vi "Email_With_Log.vi"(0 "recipients":string[](array[string]), 1 "subject ([No Subject])":string="[No Subject]", 2 "message":string, 3 "attachments":path[](array[path])) -> (5 "invalid recipients":string[](array[string]), 6 "error out":errorcluster)   [LabVIEW 2022 SP3]
uses:
  272fa2c8-f8d7-1949-8157-cfb0dd8301bf.vi
  Globals/Preference_global.vi
  Globals/Constants_global.vi
panel:
  out "Number of valid email requests":i32
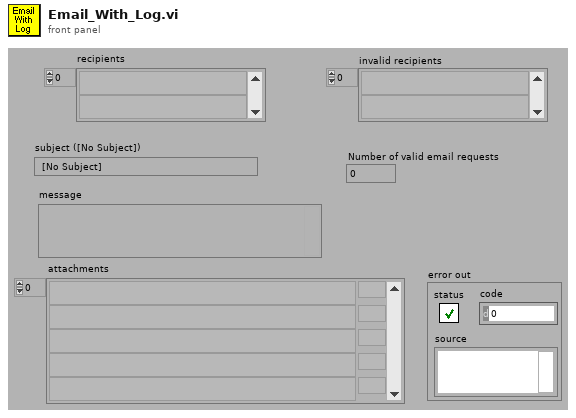
[diagram p1: front panel]
types:
  T1 = typedef "SMTPCredentials.ctl" = cluster{"User Name":string, "Password":string, "Reply to Address":string, "From Domain":string}
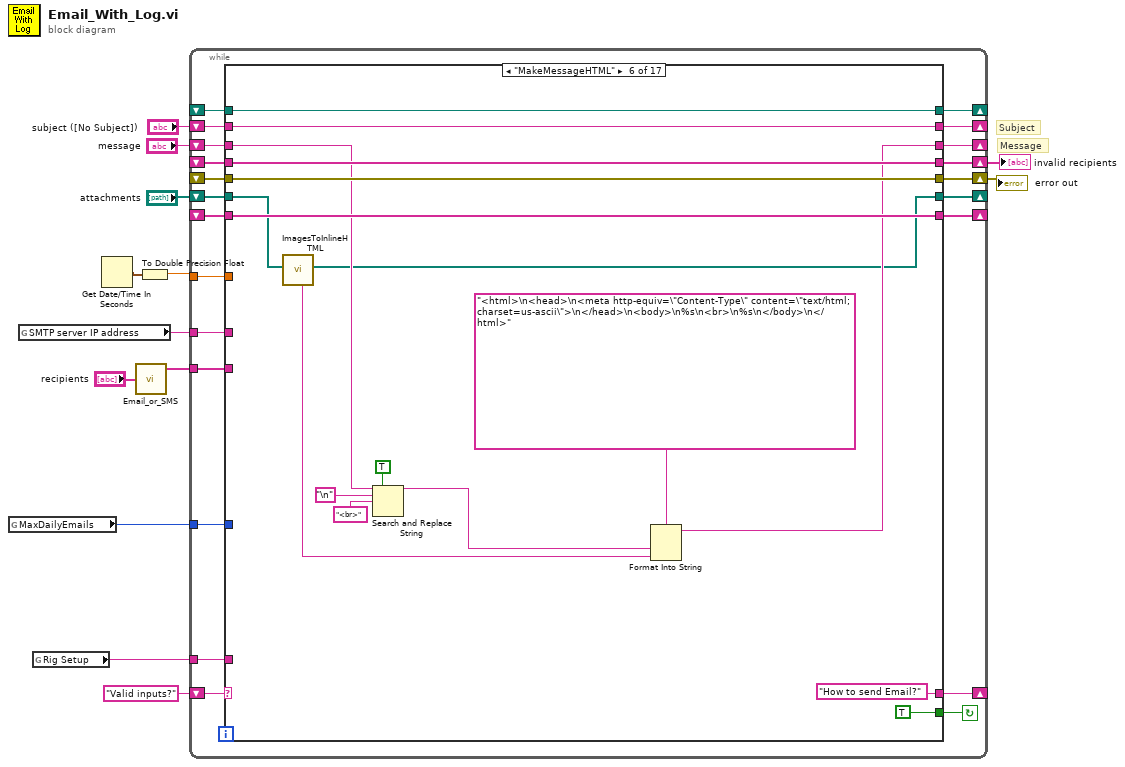
[diagram p0: block diagram]
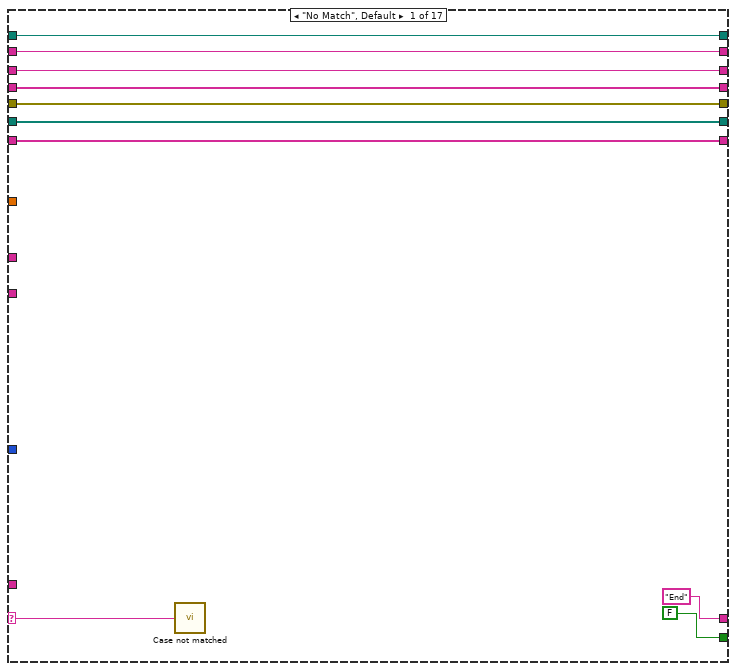
[diagram p2: hidden frame]
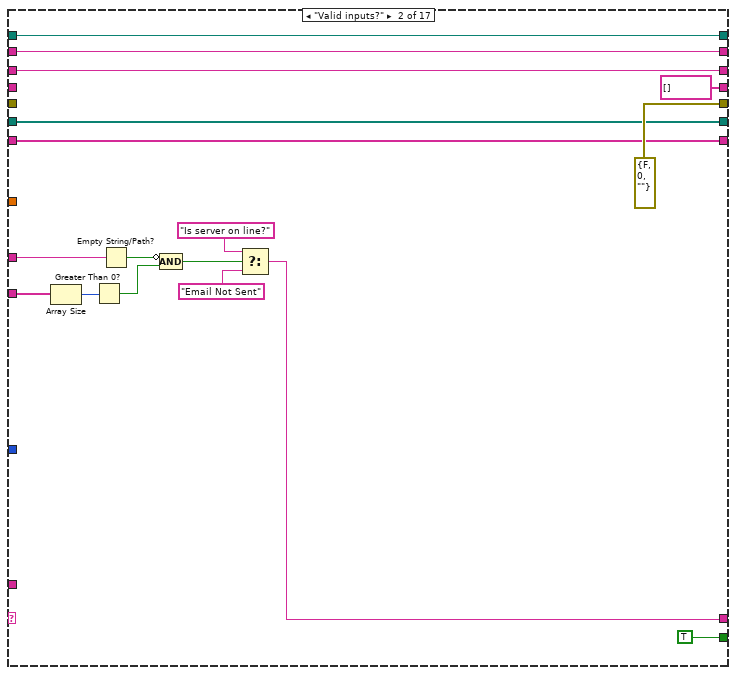
[diagram p3: hidden frame]
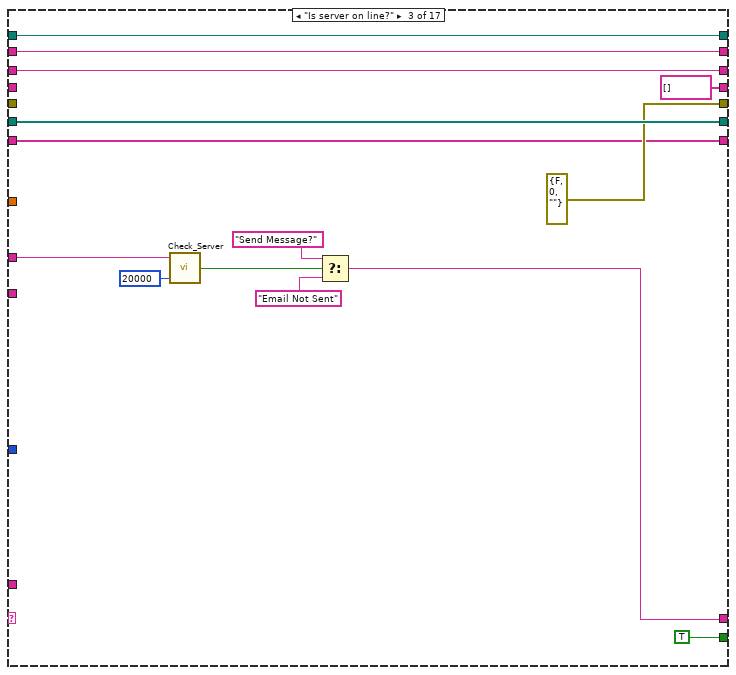
[diagram p4: hidden frame]
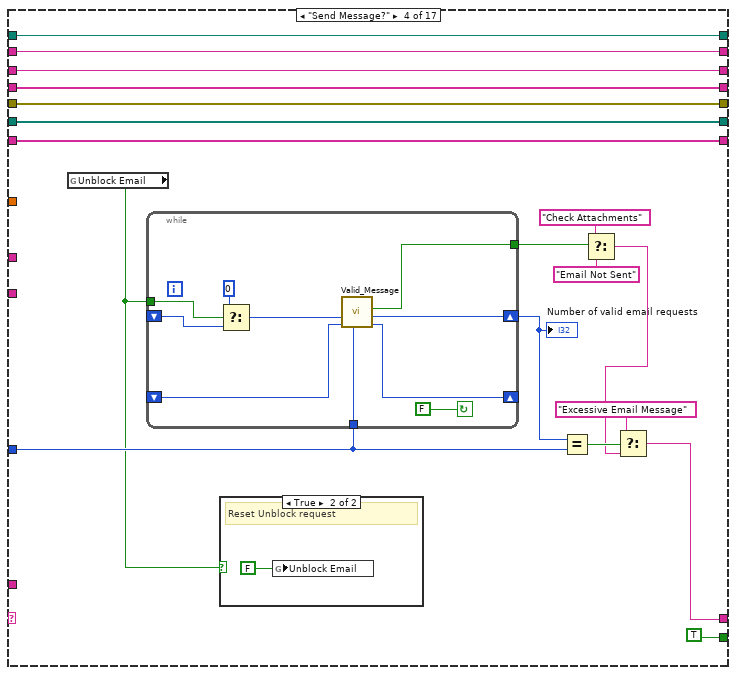
[diagram p5: hidden frame]
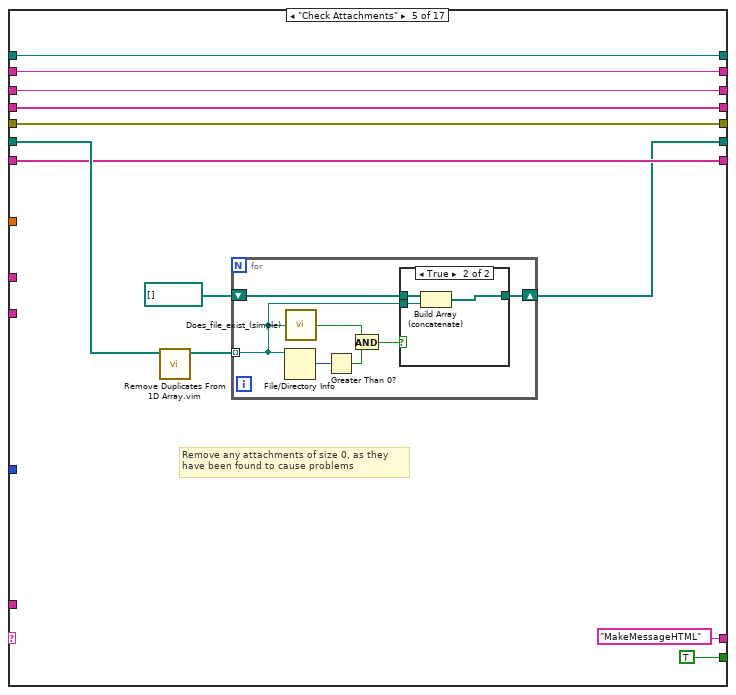
[diagram p7: hidden frame]
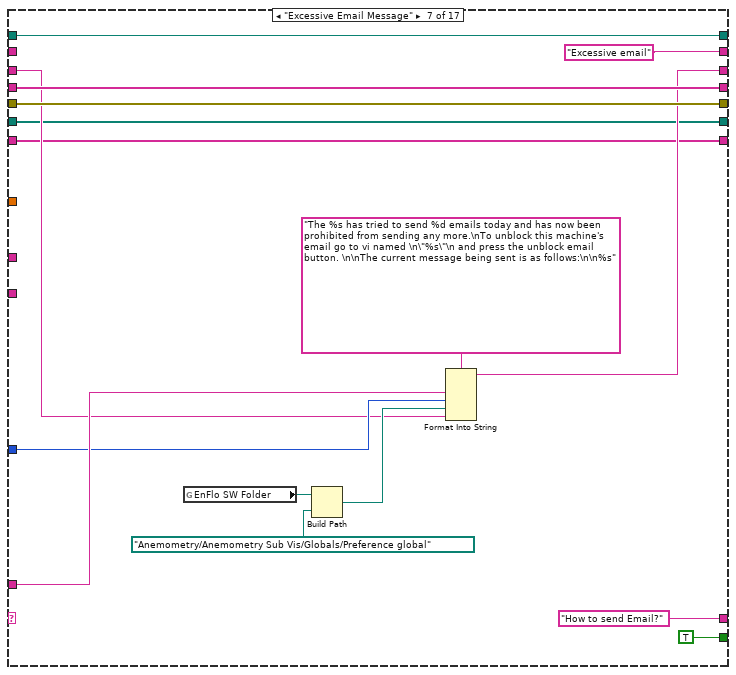
[diagram p9: hidden frame]
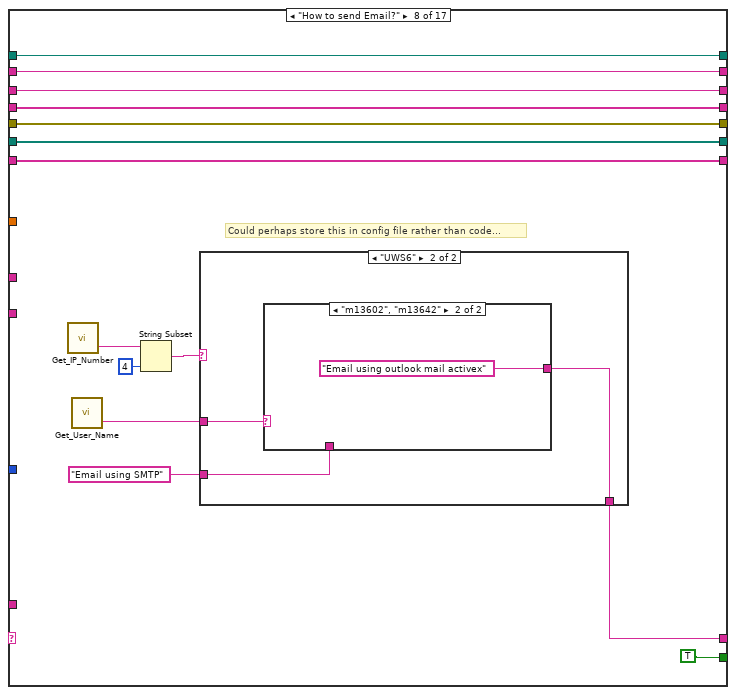
[diagram p10: hidden frame]
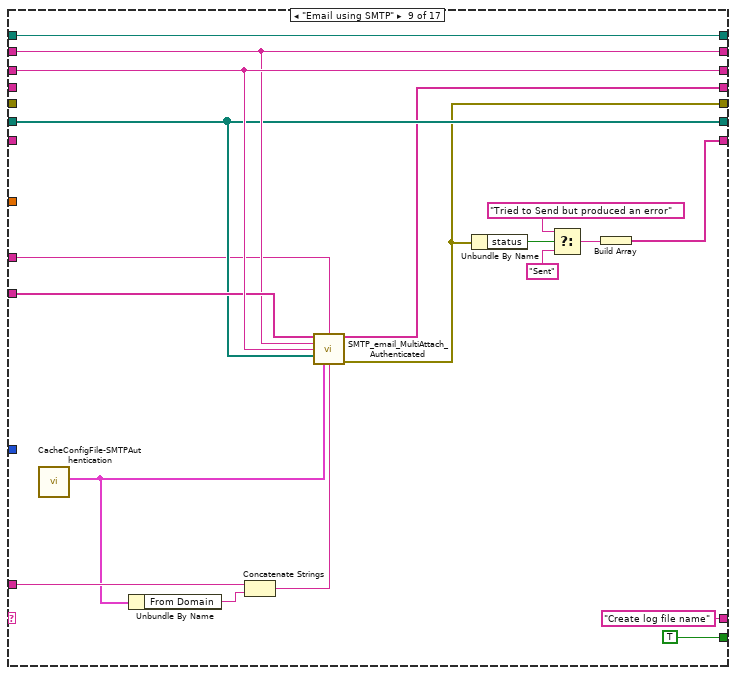
[diagram p13: hidden frame]
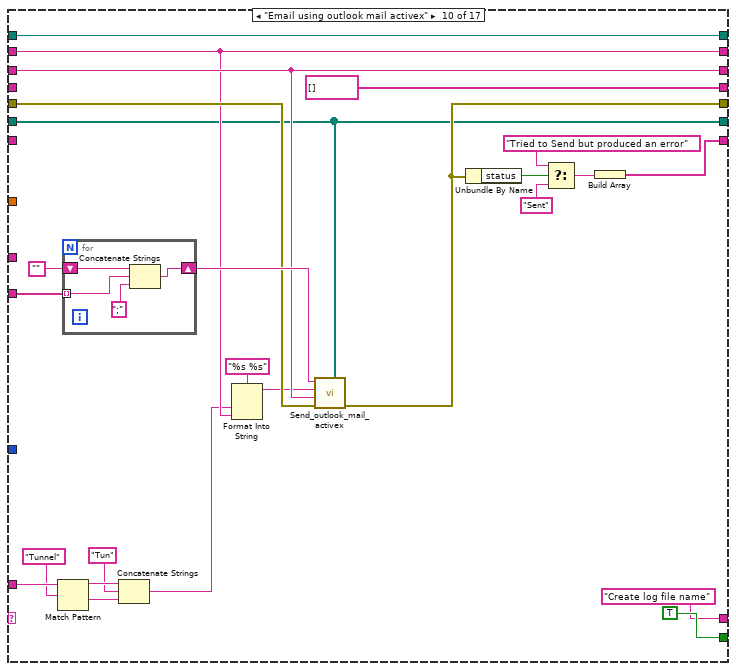
[diagram p14: hidden frame]
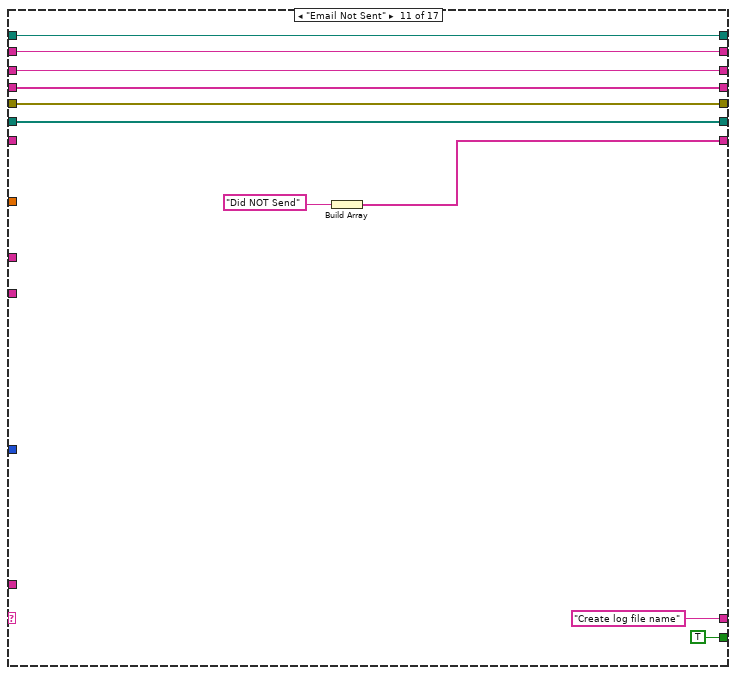
[diagram p15: hidden frame]
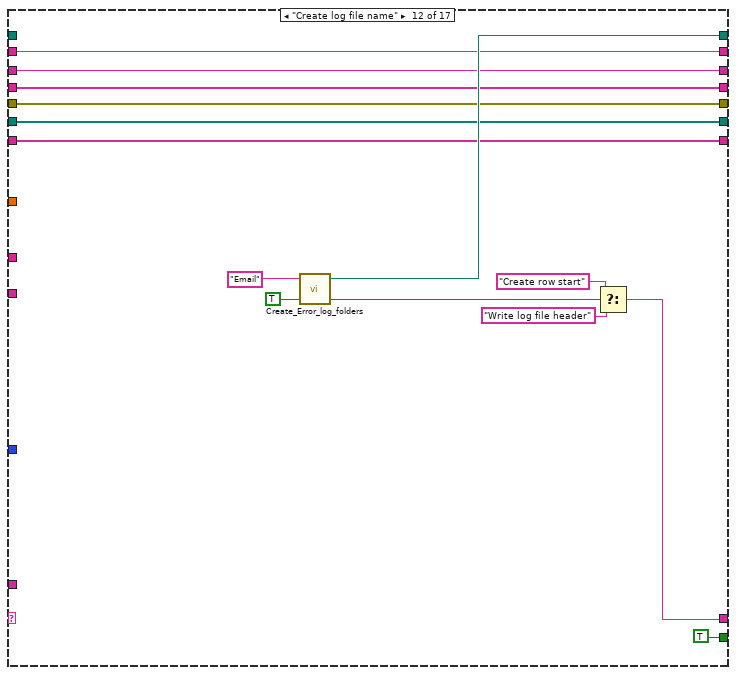
[diagram p16: hidden frame]
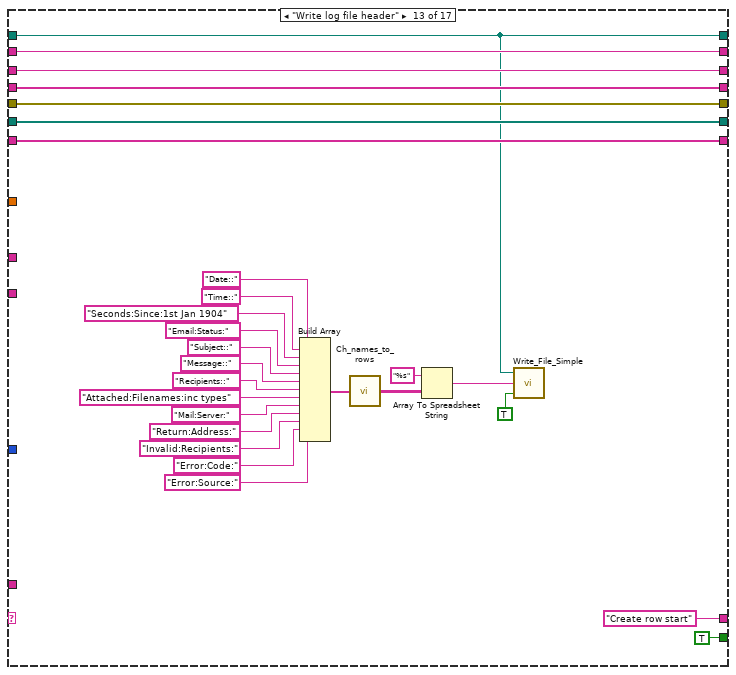
[diagram p17: hidden frame]
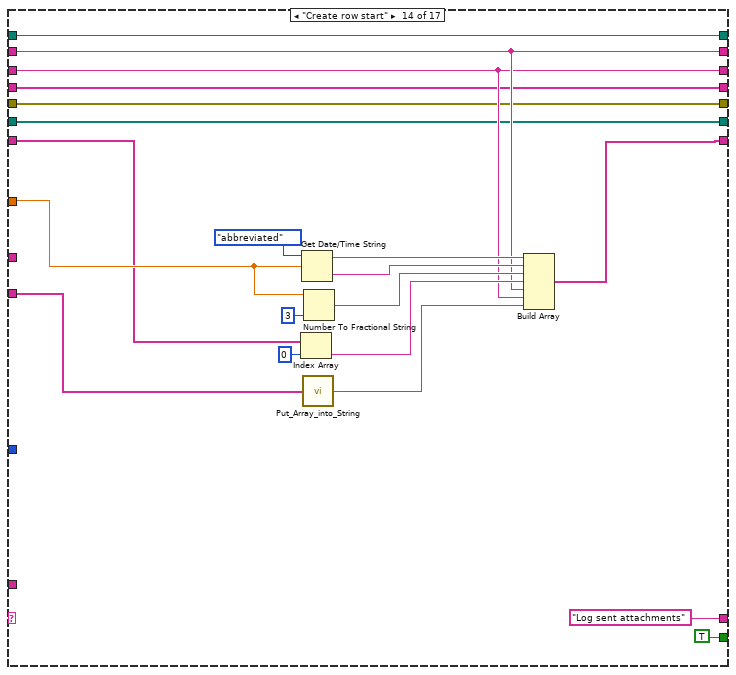
[diagram p18: hidden frame]
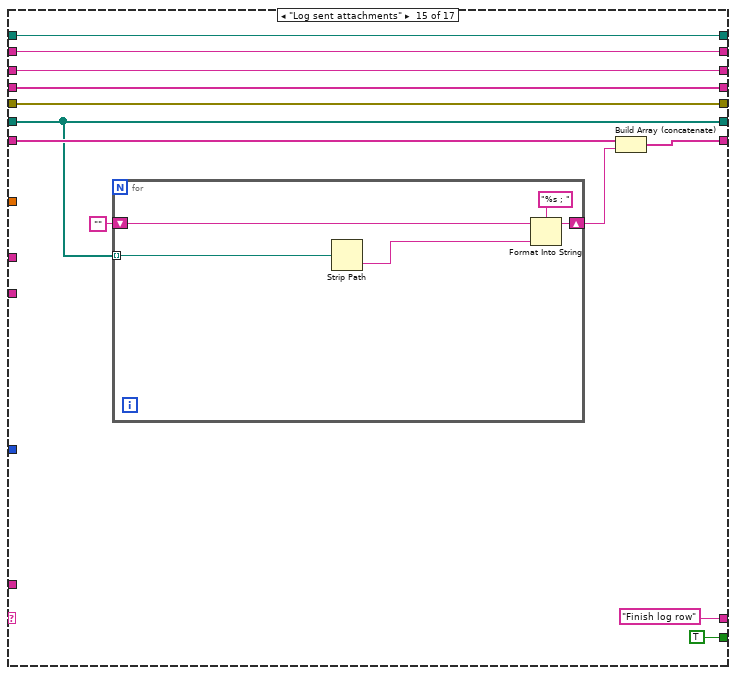
[diagram p19: hidden frame]
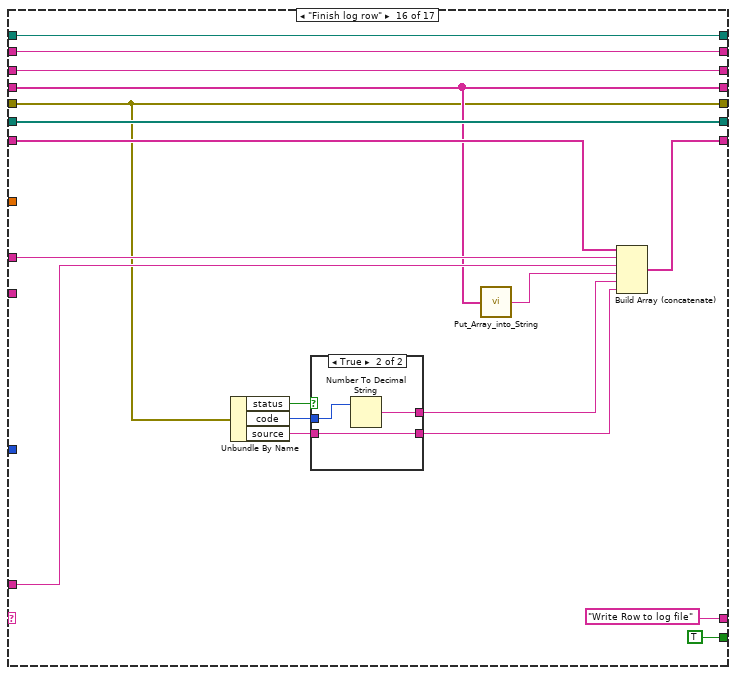
[diagram p20: hidden frame]
diagram:
  # "Message"
  # "Subject"
  n1 = global read "Preference_global.vi" "MaxDailyEmails"() -> (w1:u32)
  n2 = global read "Preference_global.vi" "SMTP server IP address"() -> (w4:string)
  n3 = global read "Preference_global.vi" "Rig Setup"() -> (w2:string)
  n4 = Get Date/Time In Seconds() -> (seconds since 1Jan1904=w12:timestamp)
  n5 = call "Email_or_SMS.vi"("Email address"="recipients") -> ("Email"=w5:string[])  [unwired: 3 out]
  n6 = To Double Precision Float(number=w12) -> (double precision float=w13:dbl)
  n7 = while {
    tunnel: w13 -> [w33]
    shift-left: "Valid inputs?" -> [w32]
    shift-right: [w34] -> _
    shift-right: [w30] -> _
    shift-left: _ -> [w31]
    tunnel: w1 -> [w29]
    shift-right: [w27] -> _
    shift-left: "subject ([No Subject])" -> [w28]
    shift-right: [w26] -> _
    shift-left: "message" -> [w25]
    shift-right: [w23] -> w9
    shift-left: _ -> [w24]
    shift-right: [w22] -> w3
    shift-left: _ -> [w21]
    tunnel: w2 -> [w20]
    shift-right: [w18] -> _
    shift-left: "attachments" -> [w19]
    tunnel: w5 -> [w17]
    tunnel: w4 -> [w16]
    shift-right: [w15] -> _
    shift-left: _ -> [w14]
    stop <- w35 continue-if-true
    n8 = case shown="\"MakeMessageHTML\"" w32 {
      selector: w32 -> [w36 _ _ _ _ _ _ _ _ _ _ _ _ _ _ _ _]
      tunnel: [FALSE ("Abort") TRUE ("Abort") TRUE ("Abort") TRUE ("Abort") TRUE ("Abort") TRUE ("Abort") TRUE ("Abort") TRUE ("Abort") TRUE ("Abort") TRUE ("Abort") TRUE ("Abort") TRUE ("status") TRUE TRUE TRUE TRUE FALSE] -> w35
      tunnel: ["End" ("f") w52 w70 w83 "MakeMessageHTML" ("f") "How to send Email?" ("f") "How to send Email?" ("f") w164 "Create log file name" ("f") "Create log file name" ("f") "Create log file name" ("f") w251 "Create row start" ("f") "Log sent attachments" ("f") "Finish log row" ("f") "Write Row to log file" ("f") "End" ("f")] -> w34
      tunnel: w33 -> [_ _ _ _ _ _ _ _ _ _ _ _ _ w295 _ _ _]
      tunnel: w31 -> [w43 w61 w75 w93 w116 w144 w160 w174 w199 w224 w238 _ w255 w292 w310 w333 w341]
      tunnel: [w43 w61 w75 w93 w116 w144 w160 w174 w199 w224 w238 w248 w255 w292 w310 w333 w341] -> w30
      tunnel: w29 -> [_ _ _ w91 _ _ w150 _ _ _ _ _ _ _ _ _ _]
      tunnel: w28 -> [w42 w48 w74 w90 w115 w143 _ w172 w195 w209 w237 w246 w268 w285 w308 w331 w348]
      tunnel: [w42 w48 w74 w90 w115 w143 "Excessive email" ("Email address") w172 w195 w209 w237 w246 w268 w285 w308 w331 w348] -> w27
      tunnel: [w41 w60 w73 w89 w114 w133 w154 w173 w198 w214 w236 w245 w267 w284 w307 w330 w347] -> w26
      tunnel: w25 -> [w41 w60 w73 w89 w114 w132 w149 w173 w198 w214 w236 w245 w267 w284 w307 w330 w347]
      tunnel: w24 -> [w40 _ _ w88 w113 w142 w159 w170 _ _ w235 w244 w266 w283 w306 w325 w346]
      tunnel: [w40 string[] [] ("invalid recipients") string[] [] ("invalid recipients") w88 w113 w142 w159 w170 w185 string[] [] ("invalid recipients") w235 w244 w266 w283 w306 w325 w346] -> w23
      tunnel: [w39 errorcluster {"status"=FALSE, "code"=0, "source"=""} ("error out") errorcluster {"status"=FALSE, "code"=0, "source"=""} ("error out") w87 w112 w141 w158 w169 w193 w212 w234 w243 w265 w282 w305 w323 w345] -> w22
      tunnel: w21 -> [w39 _ _ w87 w112 w141 w158 w169 _ w213 w234 w243 w265 w282 w305 w323 w345]
      tunnel: w20 -> [_ _ _ _ _ _ w153 _ w187 w207 _ _ _ _ _ w326 _]
      tunnel: w19 -> [w38 w46 w69 w79 w111 w131 w147 w171 w194 w201 w233 w242 w264 w281 w301 w329 w344]
      tunnel: [w38 w46 w69 w79 w106 w130 w147 w171 w194 w201 w233 w242 w264 w281 w301 w329 w344] -> w18
      tunnel: w17 -> [_ w59 _ _ _ _ _ _ w197 w216 _ _ _ w287 _ _ _]
      tunnel: w16 -> [_ w57 w65 _ _ _ _ _ w184 _ _ _ _ _ _ w327 _]
      tunnel: w14 -> [w37 w50 w67 w78 w109 w139 w146 w168 _ _ _ w241 w257 w291 w302 w328 w343]
      tunnel: [w37 w50 w67 w78 w109 w139 w146 w168 w188 w218 w230 w241 w257 w288 w309 w332 w343] -> w15
      frame "No Match", Default {
        n9 = call "Case not matched.vi"("Case Name not Matched"=w36) -> ()
      }
      frame "Valid inputs?" {
        n10 = Array Size(array=w59) -> (size(s)=w58:i32)
        n11 = Greater Than 0?(x=w58) -> (x > 0?=w56:bool)
        n12 = Empty String/Path?(string/path=w57) -> (empty?=w47:bool)
        n13 = Compound Arithmetic op=AND(invert w47, w56) -> (w55:bool)
        n14 = Select(t="Is server on line?" ("f"), s=w55, f="Email Not Sent") -> (s? t:f=w52:string)
      }
      frame "Is server on line?" {
        n15 = call "Check_Server.vi"("timeout ms (60000)"=20000, "address"=w65) -> ("OK"=w64:bool)  [unwired: 3 out]
        n16 = Select(t="Send Message?" ("f"), s=w64, f="Email Not Sent") -> (s? t:f=w70:string)
      }
      frame "Send Message?" {
        n17 = global read "Preference_global.vi" "Unblock Email"() -> (w77:bool)
        n18 = while {
          tunnel: w77 -> [w99]
          tunnel: w91 -> [w101]
          tunnel: [w102] -> w85
          shift-left: _ -> [w98]
          shift-right: [w100] -> w92
          shift-left: _ -> [w104]
          shift-right: [w103] -> _
          stop <- FALSE continue-if-true
          n19 = Select(t=0, s=w99, f=w98) -> (s? t:f=w97:i32)
          n20 = call "Valid_Message.vi"("Max per day"=w101, "day of month in"=w104, "Number of requests today In"=w97) -> ("day of month out"=w103:i32, "Number of requests today Out"=w100:i32, "Send Message"=w102:bool)  [unwired: 2 in, 4 out]
        }
        "Number of valid email requests" <- w92
        n21 = case shown="True" w77 {
          frame False {
          }
          frame True {
            # "Reset Unblock request"
            n22 = global write "Preference_global.vi" "Unblock Email"(FALSE ("Unblock Email")) -> ()
          }
        }
        n23 = Equal?(x=w92, y=w91) -> (x = y?=w86:bool)
        n24 = Select(t="Check Attachments", s=w85, f="Email Not Sent") -> (s? t:f=w84:string)
        n25 = Select(t="Excessive Email Message", s=w86, f=w84) -> (s? t:f=w83:string)
      }
      frame "Check Attachments" {
        # "Remove any attachments of size 0, as they have been found to cause problems"
        n26 = call "Remove Duplicates From 1D Array.vim"("array"=w111) -> ("array with duplicates removed"=w107:path[])  [unwired: 10 in]
        n27 = for {
          tunnel: w107 -> [w121] mode=indexing
          shift-right: [w124] -> w106
          shift-left: path[] [] -> [w123]
          n28 = File/Directory Info(path=w121) -> (size=w122:i64)  [unwired: 1 in, 6 out]
          n29 = call "Does_file_exist_(simple).vi"("Pathname"=w121) -> ("exists?"=w120:bool)
          n30 = Greater Than 0?(x=w122) -> (x > 0?=w119:bool)
          n31 = And(x=w120, y=w119) -> (x .and. y?=w118:bool)
          n32 = case shown="True" w118 {
            tunnel: [w125 w128] -> w124
            tunnel: w123 -> [w125 w127]
            tunnel: w121 -> [_ w126]
            frame False {
            }
            frame True {
              n33 = Build Array (concatenate)(w127, w126) -> (w128:path[])
            }
          }
        }
      }
      frame "MakeMessageHTML" {
        n34 = call "ImagesToInlineHTML.vi"("attachmentsIn"=w131) -> ("remainingAttachments"=w130:path[], "HTMLimgs"=w129:string)  [unwired: 8 in, 1 out]
        n35 = Search and Replace String(replace all?=TRUE ("replace all? (F)"), input string=w132, search string="\n", replace string="<br>" ("replace string (\"\")")) -> (result string=w135:string)  [unwired: 4 in, 3 out]
        n36 = Format Into String(format string="<html>\n<head>\n<meta http-equiv=\"Content-Type\" content=\"text/html; charset=us-ascii\">\n</head>\n<body>\n%s\n<br>\n%s\n</body>\n</html>", w135, w129) -> (resulting string=w133:string)  [unwired: 2 in, 1 out]
      }
      frame "Excessive Email Message" {
        n37 = global read "Constants_global.vi" "EnFlo SW Folder"() -> (w156:path)
        n38 = Build Path(base path=w156, name or relative path=path "Anemometry/Anemometry Sub Vis/Globals/Preference global") -> (appended path=w152:path)
        n39 = Format Into String(format string="The %s has tried to send %d emails today and has now been prohibited from sending any more.\nTo unblock this machine's email go to vi named \n\"%s\"\n and press the unblock email button. \n\nThe current message being sent is as follows:\n\n%s" ("Format String"), w153, w150, w152, w149) -> (resulting string=w154:string)  [unwired: 2 in, 1 out]
      }
      frame "How to send Email?" {
        # "Could perhaps store this in config file rather than code..."
        n40 = call "Get_IP_Number.vi"() -> ("bestAvailableName"=w167:string)  [unwired: 1 out]
        n41 = call "Get_User_Name.vi"() -> ("User Name"=w162:string)  [unwired: 1 in]
        n42 = String Subset(string=w167, length (rest)=4 ("length (rest)")) -> (substring=w165:string)  [unwired: 1 in]
        n43 = case shown="\"UWS6\"" w165 {
          tunnel: [w176 w178] -> w164
          tunnel: "Email using SMTP" -> [w176 w177]
          tunnel: w162 -> [_ w179]
          frame Default {
          }
          frame "UWS6" {
            n44 = case shown="\"m13602\", \"m13642\"" w179 {
              tunnel: [w180 "Email using outlook mail activex"] -> w178
              tunnel: w177 -> [w180 _]
              frame "False", Default {
              }
              frame "m13602", "m13642" {
              }
            }
          }
        }
      }
      frame "Email using SMTP" {
        n45 = call "CacheConfigFile-SMTPAuthentication.vi"() -> ("Authentication Credentials"=w182:T1)  [unwired: 11 in]
        n46 = Unbundle By Name(w182) -> ("From Domain"=w186:string)
        n47 = Concatenate Strings(w187, w186) -> (w183:string)
        n48 = call "SMTP_email_MultiAttach_Authenticated.vi"("Recipients"=w197, "SMTPServer:Port"=w184, "Subject"=w195, "Message"=w198, "Attachments"=w194, "SMTP Credentials"=w182, "From Address"=w183) -> ("invalid recipients"=w185:string[], "Error Out"=w193:errorcluster)  [unwired: 7 in]
        n49 = Unbundle By Name(w193) -> ("status"=w192:bool)
        n50 = Select(t="Tried to Send but produced an error", s=w192, f="Sent") -> (s? t:f=w189:string)
        n51 = Build Array(w189) -> (w188:string[])
      }
      frame "Email using outlook mail activex" {
        n52 = Match Pattern(string=w207, regular expression="Tunnel") -> (before substring=w205:string, after substring=w204:string)  [unwired: 1 in, 2 out]
        n53 = for {
          shift-right: [w226] -> w215
          shift-left: "" -> [w229]
          tunnel: w216 -> [w228] mode=indexing
          n54 = Concatenate Strings(w229, w228, ";") -> (w226:string)
        }
        n55 = Concatenate Strings(w205, "Tun" ("string"), w204) -> (w202:string)
        n56 = Format Into String(format string="%s %s", w202, w209) -> (resulting string=w208:string)  [unwired: 2 in, 1 out]
        n57 = call "Send_outlook_mail_activex.vi"("Attachments"=w201, "error in"=w213, "Message"=w214, "Subject"=w208, "To"=w215) -> ("error out"=w212:errorcluster)  [unwired: 6 in]
        n58 = Unbundle By Name(w212) -> ("status"=w222:bool)
        n59 = Select(t="Tried to Send but produced an error", s=w222, f="Sent") -> (s? t:f=w219:string)
        n60 = Build Array(w219) -> (w218:string[])
      }
      frame "Email Not Sent" {
        n61 = Build Array("Did NOT Send") -> (w230:string[])
      }
      frame "Create log file name" {
        n62 = call "Create_Error_log_folders.vi"("Log Filename"="Email" ("Input Element"), "Per Day Log File?"=TRUE) -> ("Local Log File"=w248:path, "exists?"=w247:bool)  [unwired: 4 in]
        n63 = Select(t="Create row start", s=w247, f="Write log file header") -> (s? t:f=w251:string)
      }
      frame "Write log file header" {
        n64 = Build Array("Date::", "Time::", "Seconds:Since:1st Jan 1904", "Email:Status:", "Subject::", "Message::", "Recipients::", "Attached:Filenames:inc types", "Mail:Server:", "Return:Address:", "Invalid:Recipients:", "Error:Code:", "Error:Source:") -> (w275:string[])
        n65 = call "Ch_names_to_rows.vi"("Channel Names"=w275) -> ("3 Row names"=w274:string[][])
        n66 = Array To Spreadsheet String(array=w274, 3:"%s" ("format string")) -> (spreadsheet string=w254:string)  [unwired: 1 out]
        n67 = call "Write_File_Simple.vi"("append to file? (new file:F)"=TRUE, "character string"=w254, "file path"=w255) -> ()  [unwired: 2 out]
      }
      frame "Create row start" {
        n68 = Index Array(array=w291, index=0) -> (element=w289:string)
        n69 = Get Date/Time String(date format (0)=enum16{"short", "long", "abbreviated"}."abbreviated", seconds (now)=w295) -> (date string=w299:string, time string=w298:string)  [unwired: 1 out]
        n70 = call "Put_Array_into_String.vi"("String array"=w287) -> ("String Value"=w286:string)
        n71 = Number To Fractional String(number=w295, precision (6)=i16 3) -> (F-format string=w294:string)  [unwired: 2 out]
        n72 = Build Array(w299, w298, w294, w289, w285, w284, w286) -> (w288:string[])
      }
      frame "Log sent attachments" {
        n73 = for {
          shift-right: [w315] -> w303
          shift-left: "" -> [w316]
          tunnel: w301 -> [w313] mode=indexing
          n74 = Strip Path(path=w313) -> (name=w317:string)  [unwired: 1 out]
          n75 = Format Into String(format string="%s ; ", initial string=w316, w317) -> (resulting string=w315:string)  [unwired: 1 in, 1 out]
        }
        n76 = Build Array (concatenate)(w302, w303) -> (w309:string[])
      }
      frame "Finish log row" {
        n77 = Unbundle By Name(w323) -> ("status"=w322:bool, "code"=w321:i32, "source"=w320:string)
        n78 = case shown="True" w322 {
          tunnel: w321 -> [_ w338]
          tunnel: w320 -> [_ w339]
          tunnel: [w336 w339] -> w319
          tunnel: [w336 w337] -> w318
          frame False {
            w336 = ""
          }
          frame True {
            n79 = Number To Decimal String(number=w338) -> (decimal integer string=w337:string)  [unwired: 1 out]
          }
        }
        n80 = call "Put_Array_into_String.vi"("String array"=w325) -> ("String Value"=w324:string)
        n81 = Build Array (concatenate)(w328, w327, w326, w324, w318, w319) -> (w332:string[])
      }
      frame "Write Row to log file" {
        n82 = for {
          shift-right: [w357] -> w349
          shift-left: "" -> [w358]
          tunnel: w343 -> [w355] mode=indexing
          n83 = call "Truncate_Excessive_Strings.vi"("String"=w355) -> ("Truncated String"=w354:string)  [unwired: 2 in]
          n84 = Concatenate Strings(w358, w354, "\t") -> (w357:string)
        }
        n85 = Concatenate Strings(w349, "\n") -> (w342:string)
        n86 = call "Write_File_Simple.vi"("append to file? (new file:F)"=TRUE, "character string"=w342, "file path"=w341) -> ()  [unwired: 2 out]
      }
    }
  }
  "invalid recipients" <- w9
  "error out" <- w3
